vi "Teleop.vi"(10 "Match Info":T1={"Autonomous Elapsed Seconds"=0.0, "TeleOp Elapsed Seconds"=0.0, "Disabled Elapsed Seconds"=0.0, "Visited Autonomous"=FALSE, "Visited TeleOp"=FALSE, "Visited Disabled"=FALSE, "Autonomous Settings"={"Autonomous Style"=enum."Independent", "VI Refnum"=refnum}}, 11 "Call Context":T2) -> ()   [LabVIEW 2017]
doc: "This VI is called for each TeleOp packet received from the DS where the robot is not disabled. It is often used to read from the joysticks and update I/O or to update setpoints for timed control loops. It should complete and return within 20 milliseconds or it may miss DS packets."
uses:
  <vilib>/Rock Robotics/WPI/DriverStation/WPI_DriverStationDerivedRobotMode.ctl
  <vilib>/Rock Robotics/WPI/DriverStation/WPI_DriverStationMatch Info.ctl
  <vilib>/Rock Robotics/WPI/Solenoid/WPI_SolenoidValue.ctl
  Change Detect.vi
  Change Detect Boolean.vi
  <vilib>/Rock Robotics/WPI/Utilities/WPI_GetSetVariantRefNum.vi
  <vilib>/Rock Robotics/Network Tables/NT Write Numeric Array.vi
  <vilib>/Rock Robotics/WPI/Solenoid/WPI_SolenoidSetEnum.vi
panel:
  out "Boolean":bool
  in  "constante":dbl=0.3 format="%#_13g"
  in  "puxa":dbl=0.6 format="%#_13g"
  in  "expele":dbl=-0.6 format="%#_13g"
  in  "negInertiaScalar":dbl=0.8
  in  "Sensitivty":dbl=1.15
  in  "WheelNonLinearity":dbl=0.65
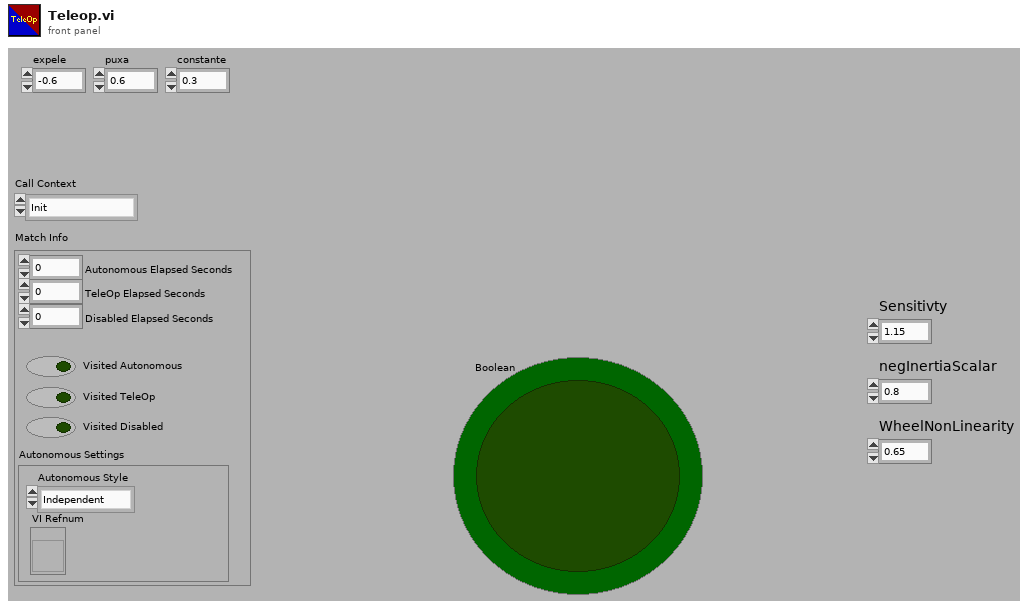
[diagram p1: front panel]
types:
  T1 = typedef "WPI_DriverStationMatch Info.ctl" = cluster{"Autonomous Elapsed Seconds":dbl, "TeleOp Elapsed Seconds":dbl, "Disabled Elapsed Seconds":dbl, "Visited Autonomous":bool, "Visited TeleOp":bool, "Visited Disabled":bool, "Autonomous Settings":cluster{"Autonomous Style":enum16{"Iterative", "Independent"}, "VI Refnum":refnum<vi>}}
  T2 = typedef "WPI_DriverStationDerivedRobotMode.ctl" = enum16{"Init", "Execute", "Stop"}
  T3 = typedef "WPI_SolenoidValue.ctl" = enum16{"Off", "On", "Forward", "Reverse"}
  T4 = typedef "WPI_JoystickDevRef.ctl" = cluster{"Device":T5}
  T5 = typedef "WPI_JoystickDeviceEnum.ctl" = enum16{"USB 0", "USB 1", "USB 2", "USB 3", "USB 4", "USB 5"}
  T6 = cluster{"Buttons[0]":bool, "Buttons[1]":bool, "Buttons[2]":bool, "Buttons[3]":bool, "Buttons[4]":bool, "Buttons[5]":bool, "Buttons[6]":bool, "Buttons[7]":bool, "Buttons[8]":bool}
  T7 = typedef "WPI_MotorControlDeviceRef.ctl" = cluster{"DeviceStatus":errorcluster, "Type":T8, "PWM":cluster{"PWM Channel":T9, "DeadBand":T10}, "CAN":cluster{"Device Number":u8, "SetOutput VI Ref":variant, "GetOutput VI Ref":variant, "Enable VI Ref":variant, "Disable VI Ref":variant, "Data":variant}, "Invert":bool, "DIO PWM":cluster{"PWM \"Enable\" Channel":T9, "DIOChannel":T11, "PWM Rate":dbl}}
  T8 = typedef "WPI_MotorControlType.ctl" = enum16{"PWM", "CAN", "DIO PWM"}
  T9 = typedef "FPGA_DIOPWMChannel.ctl" = enum8{"PWM 0", "PWM 1", "PWM 2", "PWM 3", "PWM 4", "PWM 5", "PWM 6", "PWM 7", "PWM 8", "PWM 9", "PWM MXP 0", "PWM MXP 1", "PWM MXP 2", "PWM MXP 3", "PWM MXP 4", "PWM MXP 5", "PWM MXP 6", "PWM MXP 7", "PWM MXP 8", "PWM MXP 9", "Invalid"}
  T10 = typedef "WPI_PWMDeadband.ctl" = cluster{"Name":string, "maxPositivePwm":i32, "minPositivePwm":i32, "centerPwm":i32, "maxNegativePwm":i32, "minNegativePwm":i32, "angularRange":u16}
  T11 = typedef "FPGA_DIOChannel.ctl" = enum8{"DIO 0", "DIO 1", "DIO 2", "DIO 3", "DIO 4", "DIO 5", "DIO 6", "DIO 7", "DIO 8", "DIO 9", "DIO MXP 0", "DIO MXP 1", "DIO MXP 2", "DIO MXP 3", "DIO MXP 4", "DIO MXP 5", "DIO MXP 6", "DIO MXP 7", "DIO MXP 8", "DIO MXP 9", "DIO MXP 10", "DIO MXP 11", "DIO MXP 12", "DIO MXP 13", "DIO MXP 14", "DIO MXP 15", "SPI Port CS1", "SPI Port CS2", "SPI Port CS3", "SPI Port MISO", "SPI Port MOSI", "Invalid"}
  T12 = typedef "WPI_RobotDriveDevRef.ctl" = cluster{"DevStatus":errorcluster, "Motors[]":T7[], "Square Inputs":bool, "Max Output":dbl}
  T13 = cluster{"Axes[0]":dbl, "Axes[1]":dbl, "Axes[2]":dbl, "Axes[3]":dbl, "Axes[4]":dbl, "Axes[5]":dbl, "Axes[6]":dbl, "Axes[7]":dbl, "Axes[8]":dbl}
  T14 = typedef "WPI_SwitchDevRef.ctl" = cluster{"DevStatus":errorcluster, "DIO Channel":T11, "CntIndex":T15, "Normally Closed":bool}
  T15 = typedef "FPGA_CounterCtrSystemIndex.ctl" = enum8{"Ctr 0", "Ctr 1", "Ctr 2", "Ctr 3", "Ctr 4", "Ctr 5", "Ctr 6", "Ctr 7", "Invalid"}
  T16 = typedef "WPI_SolenoidDevRef.ctl" = cluster{"DevStatus":errorcluster, "Pneumatics Control Module":u8, "Forward Solenoid Channel":T17, "Reverse Solenoid Channel":T17}
  T17 = typedef "WPI_SolenoidChannel.ctl" = enum8{"Solenoid 0", "Solenoid 1", "Solenoid 2", "Solenoid 3", "Solenoid 4", "Solenoid 5", "Solenoid 6", "Solenoid 7", "Invalid"}
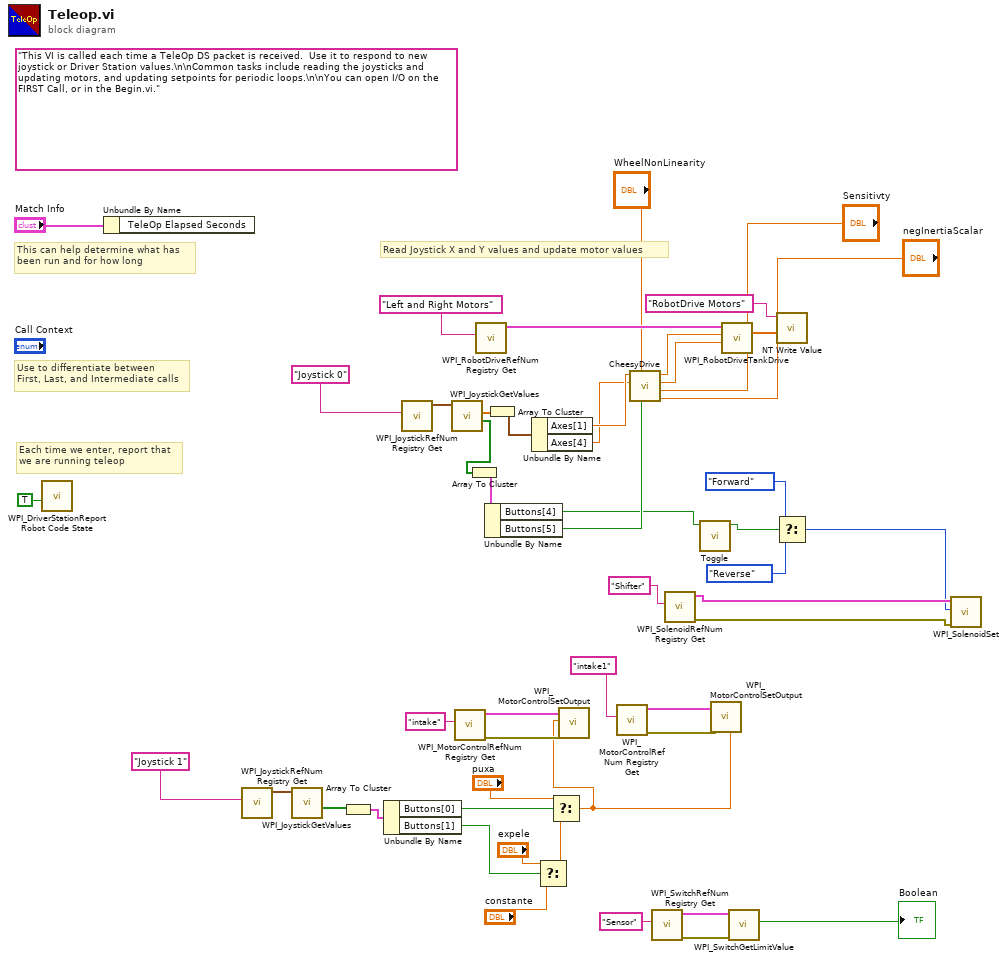
[diagram p0: block diagram]
diagram:
  (unwired) "This VI is called each time a TeleOp DS packet is received.  Use it to respond to new joystick or Driver Station values.\n\nCommon tasks include reading the joysticks and updating motors, and updating setpoints for periodic loops.\n\nYou can open I/O on the FIRST Call, or in the Begin.vi."
  # "Each time we enter, report that\nwe are running teleop"
  # "Use to differentiate between\nFirst, Last, and Intermediate calls"
  # "This can help determine what has\nbeen run and for how long"
  # "Read Joystick X and Y values and update motor values"
  n1 = call <vilib>:"WPI_DriverStationReport Robot Code State.vi"("TeleOp"=TRUE ("Autonomous")) -> ()  [unwired: 10 in, 1 out]
  n2 = Unbundle By Name("Match Info") -> ()  [unwired: 1 out]
  n3 = call <vilib>:"WPI_JoystickRefNum Registry Get.vi"("refnum name"="Joystick 1") -> ("JoystickDevRef"=w18:T4)  [unwired: 1 in, 9 out]
  n4 = call <vilib>:"WPI_JoystickGetValues.vi"("JoystickDevRef"=w18) -> ("Buttons"=w17:bool[])  [unwired: 6 in, 4 out]
  n5 = Array To Cluster(array=w17) -> (cluster=w16:T6)
  n6 = Unbundle By Name(w16) -> ("Buttons[0]"=w1:bool, "Buttons[1]"=w14:bool)
  n7 = call <vilib>:"WPI_JoystickRefNum Registry Get.vi"("refnum name"="Joystick 0") -> ("JoystickDevRef"=w45:T4)  [unwired: 1 in, 9 out]
  n8 = call <vilib>:"WPI_JoystickGetValues.vi"("JoystickDevRef"=w45) -> ("Buttons"=w35:bool[], "Axes"=w39:dbl[])  [unwired: 6 in, 3 out]
  n9 = call <vilib>:"WPI_MotorControlRefNum Registry Get.vi"("refnum name"="intake") -> ("error out"=w20:errorcluster, "MotorControlDevRef"=w21:T7)  [unwired: 9 in]
  n10 = Array To Cluster(array=w35) -> (cluster=w36:T6)
  n11 = call <vilib>:"WPI_RobotDriveRefNum Registry Get.vi"("refnum name"="Left and Right Motors") -> ("RobotDriveDevRef"=w47:T12)  [unwired: 1 in, 9 out]
  n12 = Unbundle By Name(w36) -> ("Buttons[4]"=w22:bool, "Buttons[5]"=w24:bool)
  n13 = Array To Cluster(array=w39) -> (cluster=w38:T13)
  n14 = Unbundle By Name(w38) -> ("Axes[1]"=w34:dbl, "Axes[4]"=w33:dbl)
  n15 = Select(t="expele", s=w14, f="constante") -> (s? t:f=w12:dbl)
  n16 = Select(t="puxa", s=w1, f=w12) -> (s? t:f=w7:dbl)
  n17 = call <vilib>:"WPI_MotorControlSetOutput.vi"("error in (no error)"=w20, "Output"=w7, "MotorControlDevRef"=w21) -> ()  [unwired: 6 in, 3 out]
  n18 = call <vilib>:"WPI_MotorControlRefNum Registry Get.vi"("refnum name"="intake1") -> ("error out"=w10:errorcluster, "MotorControlDevRef"=w6:T7)  [unwired: 9 in]
  n19 = call "CheesyDrive.vi"("Quickturn"=w24, "WheelNonLinearity"="WheelNonLinearity", "negInertiaScalar"="negInertiaScalar", "Sensitivty"="Sensitivty", "Wheel"=w33, "Throttle"=w34) -> ("Right PWM"=w40:dbl, "Left PWM"=w41:dbl)  [unwired: 4 in]
  n20 = call <vilib>:"WPI_SwitchRefNum Registry Get.vi"("refnum name"="Sensor") -> ("error out"=w4:errorcluster, "SwitchDevRef"=w5:T14)  [unwired: 9 in]
  n21 = call <vilib>:"WPI_SolenoidRefNum Registry Get.vi"("refnum name"="Shifter") -> ("error out"=w28:errorcluster, "SolenoidDevRef"=w29:T16)  [unwired: 9 in]
  n22 = call "Toggle.vi"("In"=w22) -> ("Toggled"=w23:bool)  [unwired: 10 in]
  n23 = call <vilib>:"WPI_MotorControlSetOutput.vi"("error in (no error)"=w10, "Output"=w7, "MotorControlDevRef"=w6) -> ()  [unwired: 6 in, 3 out]
  n24 = call <vilib>:"WPI_RobotDriveTankDrive.vi"("Right axis value"=w40, "Left axis value"=w41, "RobotDriveDevRef"=w47) -> ("Motor Values"=w43:dbl[])  [unwired: 6 in, 2 out]
  n25 = call <vilib>:"WPI_SwitchGetLimitValue.vi"("error in (no error)"=w4, "SwitchDevRef"=w5) -> ("Switch Pressed"=→"Boolean":bool)  [unwired: 7 in, 2 out]
  n26 = call-poly <vilib>:"NT Write Value.vi"("Numeric Array"=w43, "Name"="RobotDrive Motors") -> ()  [unwired: 9 in, 1 out]
  n27 = Select(t=WPI_SolenoidValue."Forward" ("Value"), s=w23, f=WPI_SolenoidValue."Reverse" ("Value")) -> (s? t:f=w25:T3)
  n28 = call-poly <vilib>:"WPI_SolenoidSet.vi"("error in (no error)"=w28, "Value"=w25, "SolenoidDevRef"=w29) -> ()  [unwired: 7 in, 2 out]
